vi "trajectory tracking.vi"() -> ()   [LabVIEW 2018]
doc: "Demonstrates the use of the Network Streams functions to send LED status to the myRIO target."
uses:
  <vilib>/addons/zeromq/socket_type.ctl
  <vilib>/ErrorRing/Error Ring.xnode
  <vilib>/vision/NI_Vision_Development_Module.lvlib
  <vilib>/addons/zeromq/zmq_socket.lvclass
  <vilib>/addons/zeromq/zmq_context.lvclass
  <vilib>/addons/zeromq/zeromq.lvlib
panel:
  out "u(t)_y":ext
  out "u(t)_x":ext
  out "relative_real_y_color":ext
  out "relative_real_x_color":ext
  in  "中心轨迹":bool
  in  "打开彩色点轨迹":bool
  out "relative_real_y_color":ext
  out "relative_real_x_color":ext
  out "彩色轨迹":T1(plugin-control)
  out "end_point_y":ext
  out "end_point_x":ext
  out "cy":ext
  out "cx":ext
  out "c":ext
  in  "簇 10":T2={"c"=100000.0, "cx"=100000.0, "cy"=100000.0, "start_point_x"=100000.0, "start_point_y"=100000.0}
  out "输出簇":T3
  in  "簇 9":T3={"a"=[], "b"=1.0, "a2"=[], "left1"=1.0, "top1"=1.0, "left2"=1.0, "top2"=1.0, "delta1"=1.0, "delta2"=1.0}
  in  "delta2":dbl=100.0
  out "bottom2":dbl
  out "right2":dbl
  out "top2":dbl
  out "left2":dbl
  in  "delta1":dbl=100.0
  out "bottom1":dbl
  out "right1":dbl
  out "top1":dbl
  out "left1":dbl
  out "delta_pr":dbl
  out "delta_dr":dbl
  in  "k2":dbl=-0.3
  in  "K1":dbl=0.3
  in  "Operation":T4(ring)=enum."Erode"
  out "old_real_relative_point_y":dbl
  out "old_real_relative_point_x":dbl
  out "real_relative_start_point_y":dbl
  out "real_relative_start_point_x":dbl
  out "Bounding Box.Y Top 2":i32
  out "Bounding Box.X Left 2":i32
  out "Ki part":dbl
  out "Kd part":dbl
  out "Kp part":dbl
  out "Ki part":dbl
  out "Kd part":dbl
  out "Kp part":dbl
  in  "Ki":dbl=0.0033
  in  "Kd":dbl=1e-05
  in  "Kp":dbl=0.01
  in  "Ki":dbl=0.0033
  in  "Kd":dbl=1e-05
  in  "Kp":dbl=0.01
  out "添加的数组":dbl[](array[numeric])
  out "desired_relative_point_y":dbl=820.0
  out "desired_relative_point_x":dbl=730.0
  out "MLP_pr":dbl=20.0
  out "MLP_dr":dbl=8.0
  out "error_relative_point_y":dbl
  out "error_relative_point_x":dbl
  out "real_relative_end_point_y":dbl
  out "real_relative_end_point_x":dbl
  out "magnet_input_pr":dbl
  out "magnet_input_dr":dbl
  in  "打开仅尖端轨迹":bool
  out "仅尖端轨迹":T1(plugin-control)
  out "Bounding Box.Y Top":i32
  out "Bounding Box.X Left":i32
  out "curve_min_y":dbl
  out "curve_min_x":dbl
  out "curve_max_y":dbl
  out "curve_max_x":dbl
  out "relative_end_point_y":dbl
  out "relative_end_point_x":dbl
  out "delta_y":dbl
  out "delta_x":dbl
  out "pr":dbl=-28.0
  out "tan(v)":dbl
  out "delta_velocity":dbl format="%#_10g"
  out "delta_time":dbl
  out "now time":timestamp[](array[timestamp])
  out "prev time":timestamp[](array[timestamp])
  out "delta_distance":dbl
  out "prev_end_point_y":dbl
  out "prev_end_point_x":dbl
  out "now_end_point_y":dbl
  out "now_end_point_x":dbl
  out "prev_end_point_y":dbl[](array[numeric])
  out "prev_end_point_x":dbl[](array[numeric])
  out "dr":dbl=120.0
  in  "Ar":sgl=11.0
  out "all parameters":dbl[][](array[numeric])
  out "direction angle":sgl[](array[numeric])
  out "dr":sgl
  out "strength":dbl[](array[numeric])
  out "场强":dbl
  out "end_point_y":T5
  out "end_point_x":dbl[](array[numeric])
  out "start_point_y":dbl[](array[numeric])
  out "start_point_x":dbl[](array[numeric])
  out "T":i32[](array[numeric])
  out "c":dbl[](array[numeric])
  out "b":dbl[](array[numeric])
  out "a\na":dbl[](array[numeric])
  out "c":dbl
  out "b":dbl
  out "a":dbl
  out "Angles (deg)":sgl[](array[numeric]) format="%.2f"
  in  "wr":sgl
  in  "打开轨迹":bool
  out "中心轨迹和尖端轨迹":T1(plugin-control)
  out "end_y":dbl
  out "end_x":dbl
  out "start_y":dbl
  out "start_x":dbl
  out "Image Pixels (U8)":u8[][](array[numeric])
  in  "Poly":dbl
  out "中心轨迹":T1(plugin-control)
  in  "保存按钮":bool
  out "Object Center":cluster{"X":sgl, "Y":sgl}
  out "黑白图":T1(plugin-control)
  in  "Number of Erosion":i32=5
  in  "Settings":T6={"Objects"=1, "Threshold"=128, "Reject Border"=FALSE, "Fill Holes"=FALSE, "Min Object Size"=TRUE, "Min Size"=1700, "Max Object Size"=FALSE, "Max Size"=100, "Show Search Area"=TRUE, "Show Center"=TRUE, "Show Bounding Box"=TRUE} {"Objects" items=["Bright Objects", "Dark Objects"]; "Threshold" min=1 max=999999999 step=1; "Max Size" min=1 max=999999999 step=1; "Min Size" min=1 max=999999999 step=1}
  out "Objects":T7(array[cluster]) {"Aspect Ratio" format="%.2f"; "Orientation" format="%.2f"; "Area" format="%.2f"; "Object Center"."Y" format="%.2f"; "Object Center"."X" format="%.2f"}
  in  "Search Rect (entire image)":T8={"Left"=350, "Top"=150, "Right"=1050, "Bottom"=1080, "Rotation"=0.0} {"Rotation" format="%.2f"; "Left" scale=0.0..1024.0; "Right" scale=0.0..1024.0}
  in  "Range":cluster{"Lower value":sgl, "Upper value":sgl}={"Lower value"=182.0, "Upper value"=255.0} {"Upper value" format="%.2f"; "Lower value" format="%.2f"}
  out "原图":T1(plugin-control)
  in  "停止":bool
  out "T":i32
  out "T":i32
  in  "磁场变换":bool=TRUE
  in  "Pause":bool
  out "Array":ext[](array[numeric])
  in  "Parameter Settings":T9(tab)=enum."Rotating Field" caption="Field Types"
  in  "Ag":dbl
  in  "dg":dbl
  in  "pg":dbl
  in  "fg":dbl
  in  "AoOF":dbl
  in  "fo":sgl
  in  "do":sgl
  in  "oo":sgl
  in  "po":sgl
  in  "cc":sgl
  in  "pc":sgl
  in  "wc":sgl
  in  "dc":sgl
  in  "Ac":dbl
  in  "Dis phase step":dbl
  in  "Dis phase frequency (Hz)":dbl
  in  "Dis tumbling frequency (Hz)":dbl
  in  "Dis strength(mT)":dbl
  in  "Swa strength (mT)":dbl
  in  "Swa frequency (Hz)":dbl
  in  "Swa pitch angle (deg)":dbl
  in  "Swa direction angle (deg)":dbl
  in  "Swa ratio":dbl=1.0
  in  "Pitch Angle (rotating around Constant, deg)":dbl
  in  "Ratio (A/C)":sgl
  in  "Direction Angle (deg)":sgl
  in  "Pitch Angle (rotating around Origin, deg)":sgl
  in  "Frequency (Hz)":sgl
  in  "Strength (mT)":dbl
  in  "Ar 2":dbl caption="Ar"
  in  "ratio":sgl
  in  "pr  2":sgl
  in  "dr  2":sgl
  in  "wr  2":sgl
  in  "p_x":sgl
  out "Numeric 5":i32
  in  "Stop":bool
  out "error out":errorcluster
  in  "Target IP Address":string="172.22.11.2"
  # "Overview: Magnetic field calculation, and send parameters to myRIO\nInstructions:\n1. Verify the value of Target IP Address. Set Visa resource name.\n2. Ensure RT Main.vi is already running. \n3. Run this VI. Set parameters of magnetic field."
  # "Strength (mT)"
  # "Frequency (Hz)"
  # "Pitch Angle (deg)"
  # "Direction Angle (deg)"
  # "Strength (mT)"
  # "Pitch Angle (deg)"
  # "Direction Angle (deg)"
  # "Frequency (Hz)"
  # "Strength (mT)"
  # "Oscilation Frequency (Hz)"
  # "Oscilation Angle (deg)"
  # "Pitch Angle (deg)"
  # "Direction Angle (deg)"
  # "Strength (mT)"
  # "Frequency (Hz)"
  # "Pitch Angle (deg)"
  # "Direction Angle (deg)"
  # "Conical Angle (deg)"
  # "Strength (mT)"
  # "Tumbling Frequency (Hz)"
  # "Phase Frequency (Hz)"
  # "Phase Step"
  # "Strength (mT)"
  # "Frequency (Hz)"
  # "Pitch Angle (deg)"
  # "Direction Angle (deg)"
  # "Ratio"
  # "Strength (mT)"
  # "Frequency (Hz)"
  # "Ratio (A/C)"
  # "Direction Angle (deg)"
  # "Pitch Angle (rotating around Origin, deg)"
  # "Pitch Angle (rotating around Constant, deg)"
  # "Strength (mT)"
  # "Frequency (Hz)"
  # "Pitch Angle Y (deg)"
  # "Pitch Angle X (deg)"
  # "Direction Angle (deg)"
  # "ratio (l/s)"
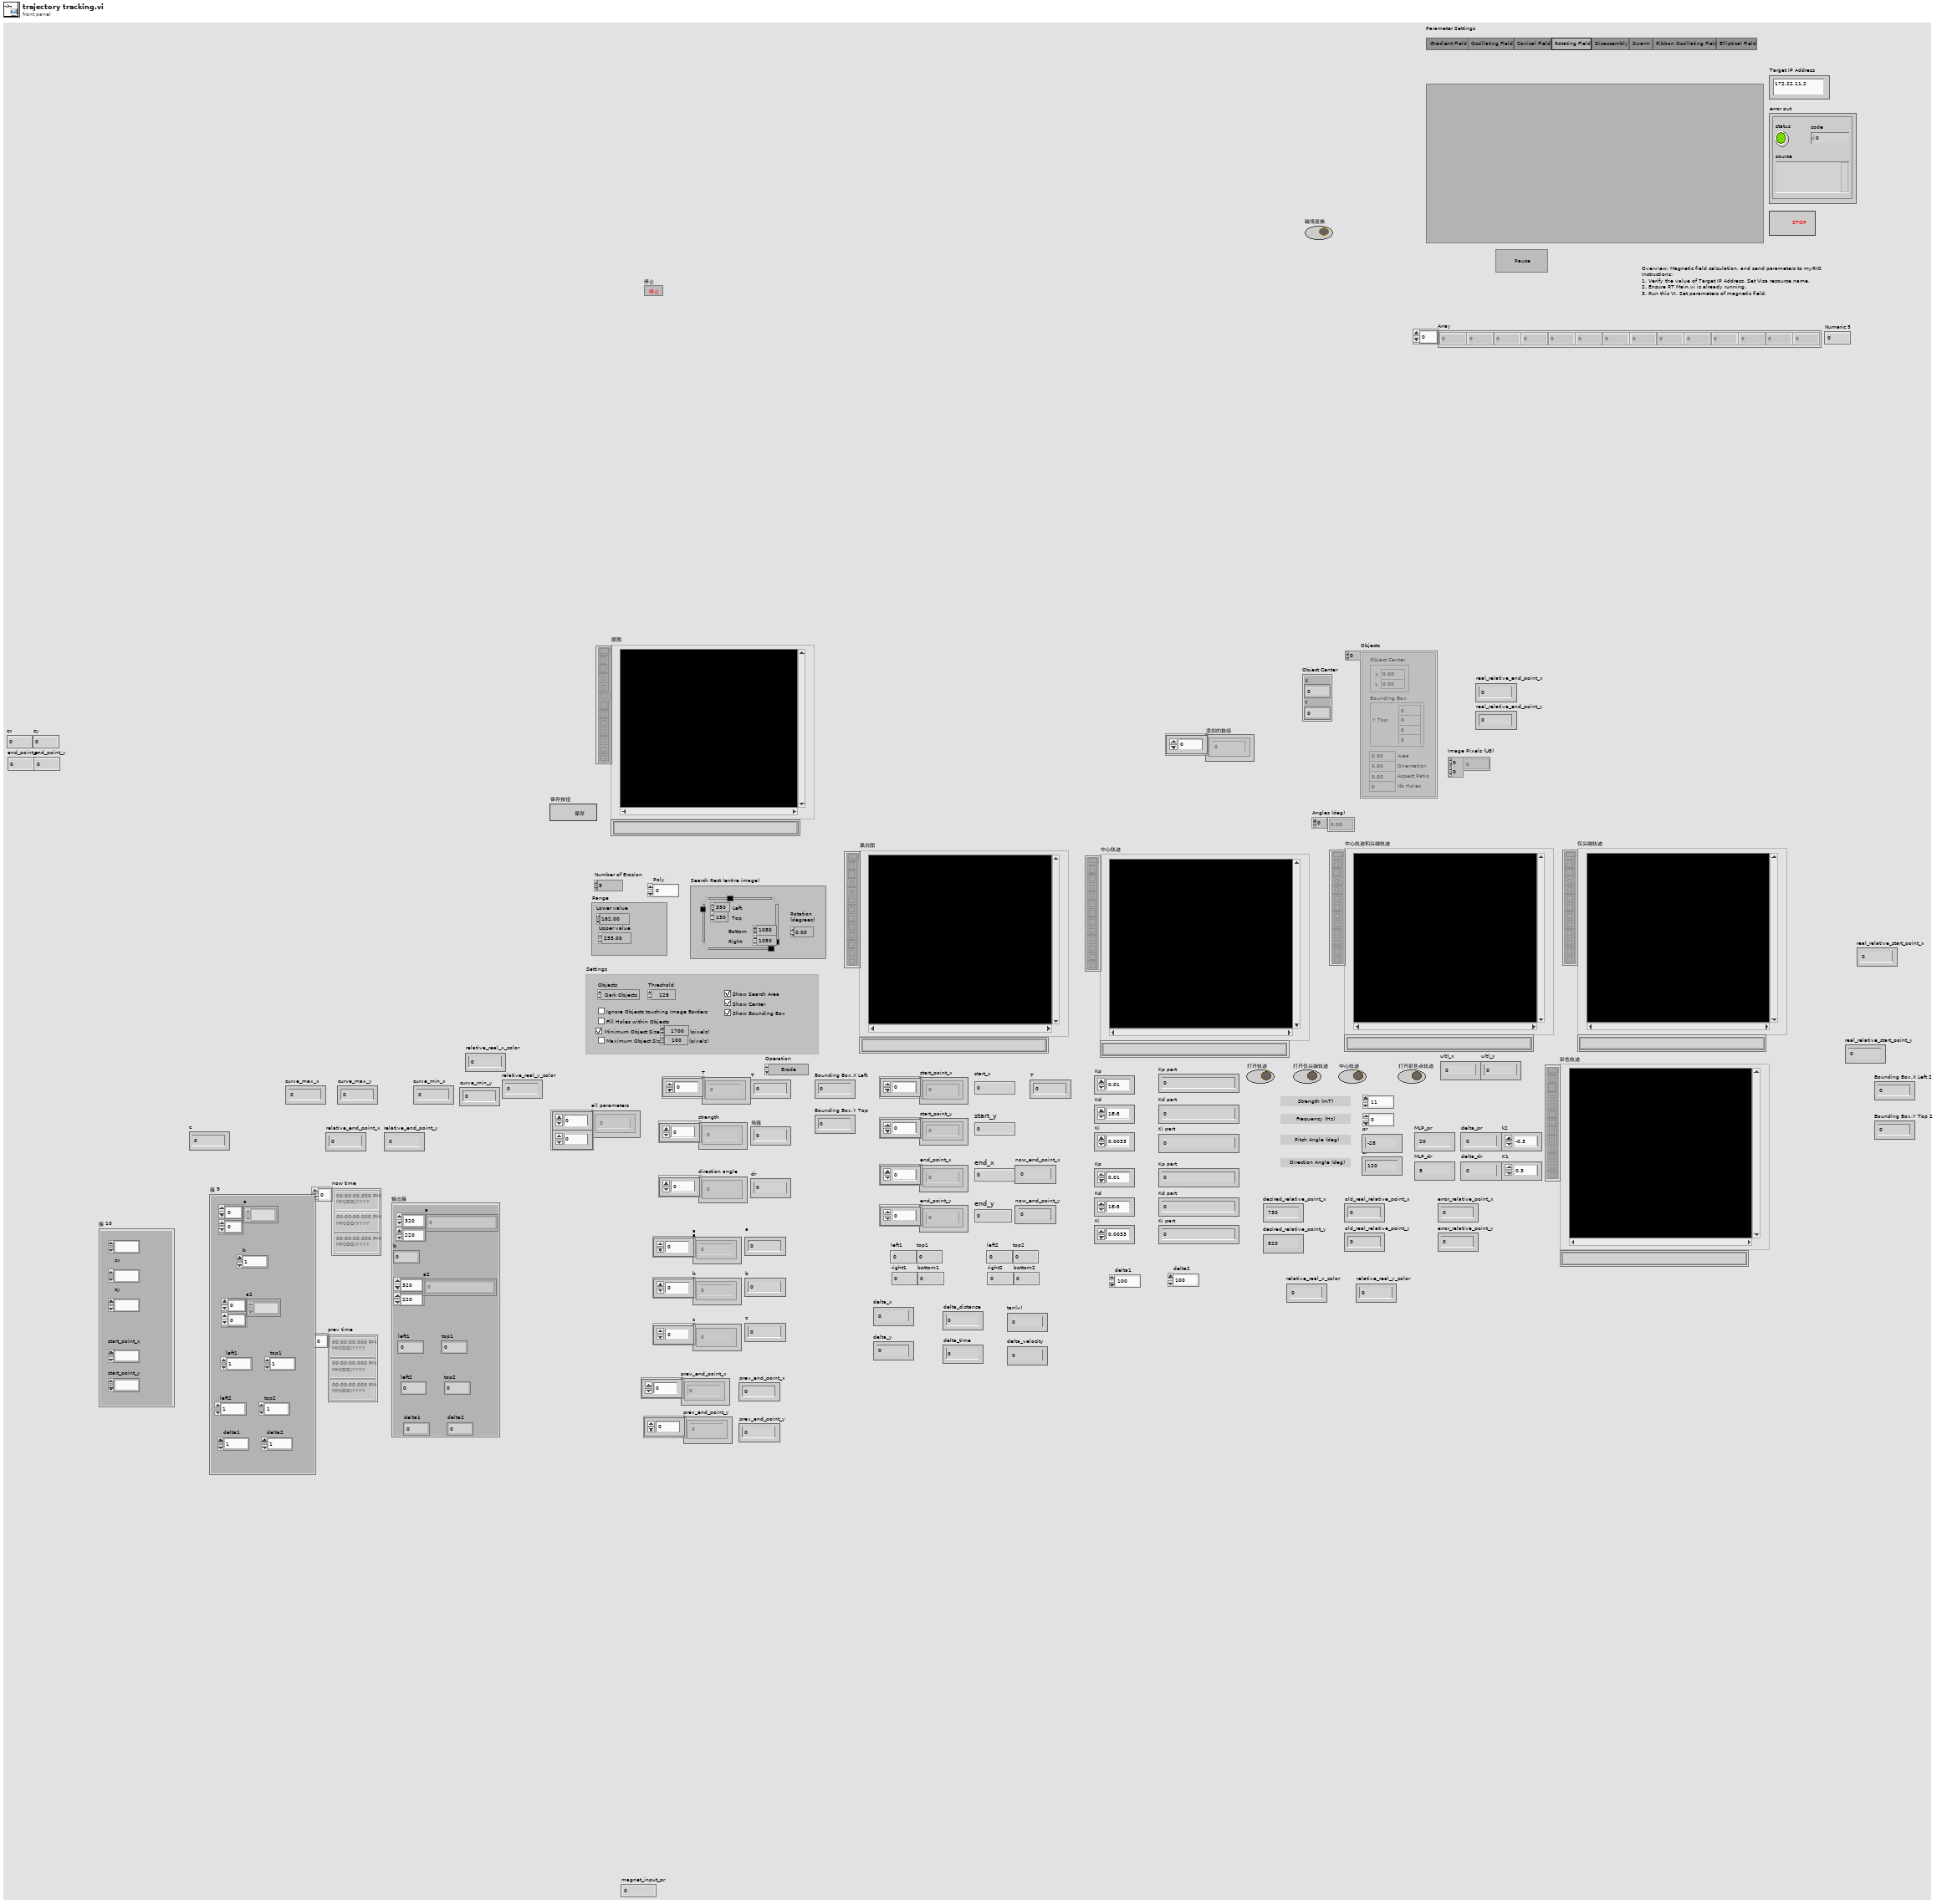
[diagram p1: front panel]
types:
  T1 = typedef "IMAQ Image.ctl" = refnum<image>
  T2 = cluster{"c":ext, "cx":ext, "cy":ext, "start_point_x":ext, "start_point_y":ext}
  T3 = cluster{"a":ext[][], "b":dbl, "a2":ext[][], "left1":dbl, "top1":dbl, "left2":dbl, "top2":dbl, "delta1":dbl, "delta2":dbl}
  T4 = enum32{"AutoM", "Close", "Dilate", "Erode", "Gradient", "Gradient in", "Gradient out", "HitMiss", "Open", "PClose", "POpen", "Thick", "Thin"}
  T5 = typedef "控件 3.ctl" = dbl[]
  T6 = cluster{"Objects":u16, "Threshold":i32, "Reject Border":bool, "Fill Holes":bool, "Min Object Size":bool, "Min Size":i32, "Max Object Size":bool, "Max Size":i32, "Show Search Area":bool, "Show Center":bool, "Show Bounding Box":bool}
  T7 = cluster{"Object Center":cluster{"X":sgl, "Y":sgl}, "Bounding Box":cluster{"X Left":i32, "Y Top":i32, "X Right":i32, "Y Bottom":i32}, "Area":sgl, "Orientation":sgl, "Aspect Ratio":sgl, "Nb Holes":i32}[]
  T8 = typedef "IMAQ Rectangle" = cluster{"Left":i32, "Top":i32, "Right":i32, "Bottom":i32, "Rotation":dbl}
  T9 = enum32{"Gradient Field ", "Oscillating Field", "Conical Field", "Rotating Field", "Disassembly", "Swarm", "Ribbon Oscillating Field", "Elliptical Field"}
  T10 = typedef "zeromq.lvlib/socket_type.ctl" = enum8{"ZMQ_PAIR", "ZMQ_PUB", "ZMQ_SUB", "ZMQ_REQ", "ZMQ_REP", "ZMQ_DEALER", "ZMQ_ROUTER", "ZMQ_PULL", "ZMQ_PUSH", "ZMQ_XPUB", "ZMQ_XSUB", "ZMQ_STREAM", "ZMQ_SERVER", "ZMQ_CLIENT", "ZMQ_RADIO", "ZMQ_DISH", "ZMQ_GATHER", "ZMQ_SCATTER", "ZMQ_DGRAM"}
  T11 = typedef "Image Type" = u32
  T12 = cluster{"Object Center":cluster{"X":sgl, "Y":sgl}, "Bounding Box":cluster{"X Left":i32, "Y Top":i32, "X Right":i32, "Y Bottom":i32}, "Area":sgl, "Orientation":sgl, "Aspect Ratio":sgl, "Nb Holes":i32}
  T13 = cluster{"X Left":i32, "Y Top":i32, "X Right":i32, "Y Bottom":i32, "Rotation":dbl}
  T14 = typedef "ROI Descriptor" = cluster{"Global Rectangle":i32[], "Contours":cluster{"ID":enum32{"External", "Internal"}, "Type":u32, "Coordinates":i32[]}[]}
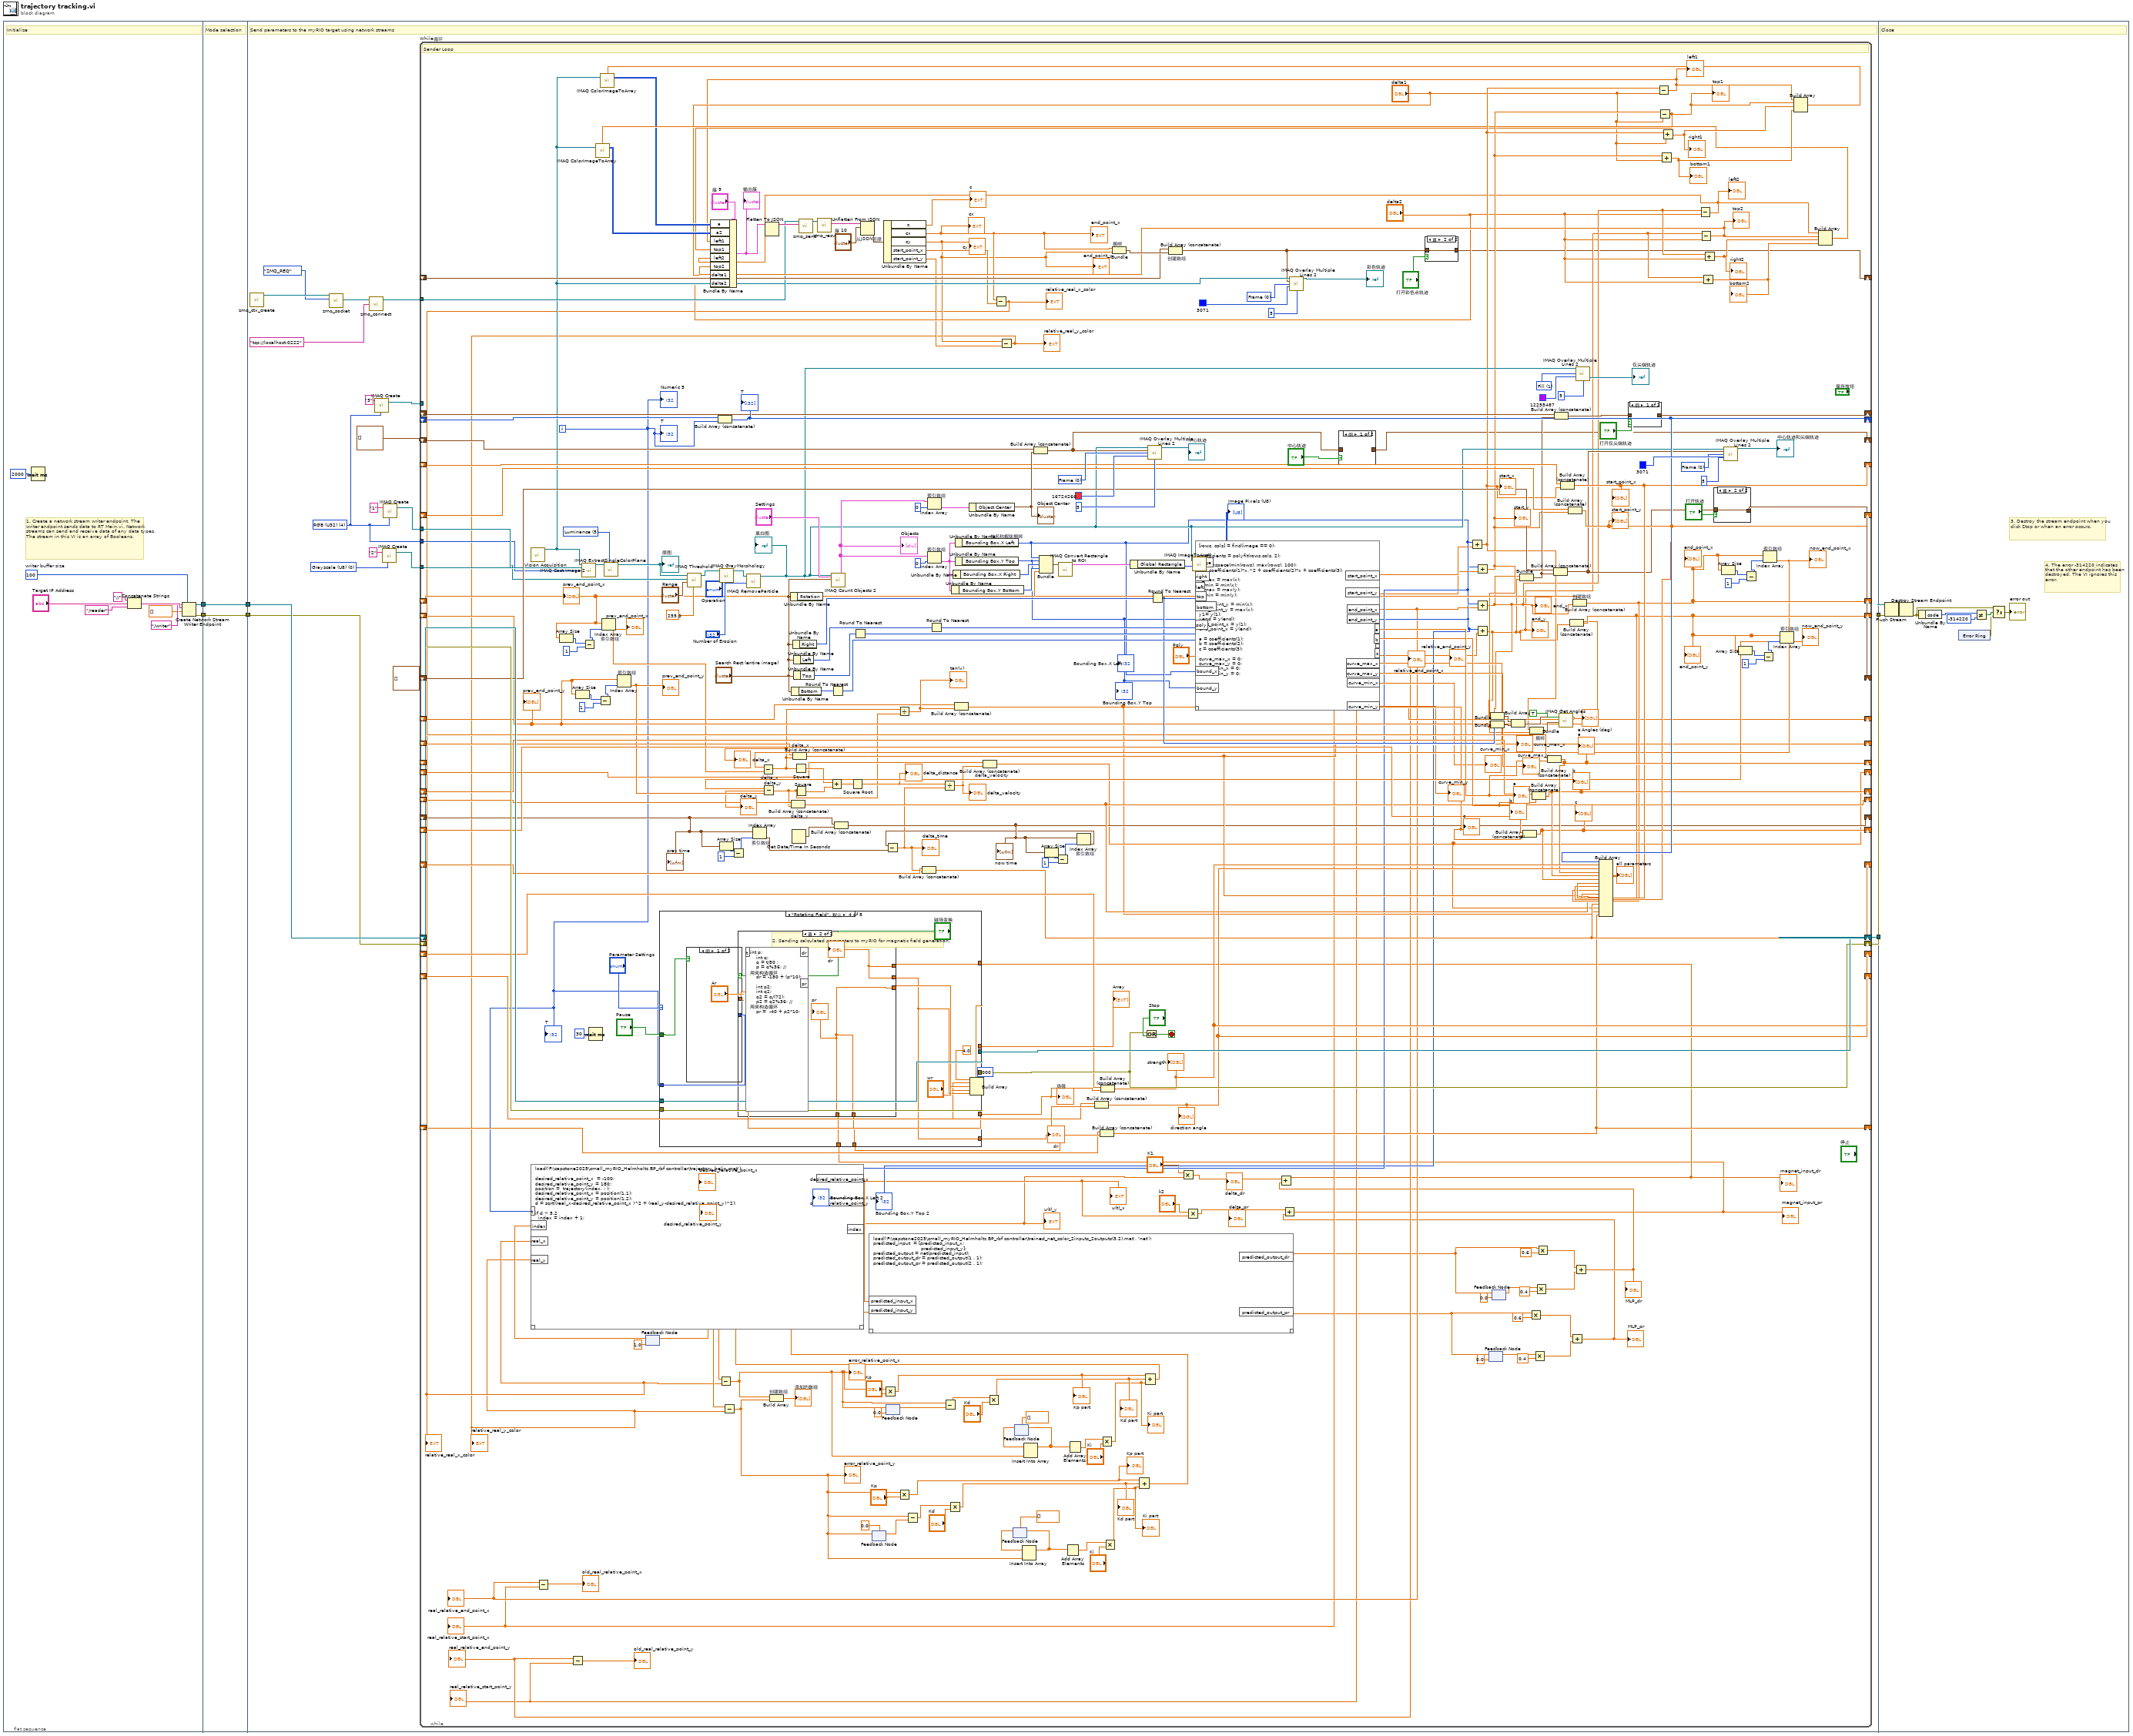
[diagram p0: block diagram]
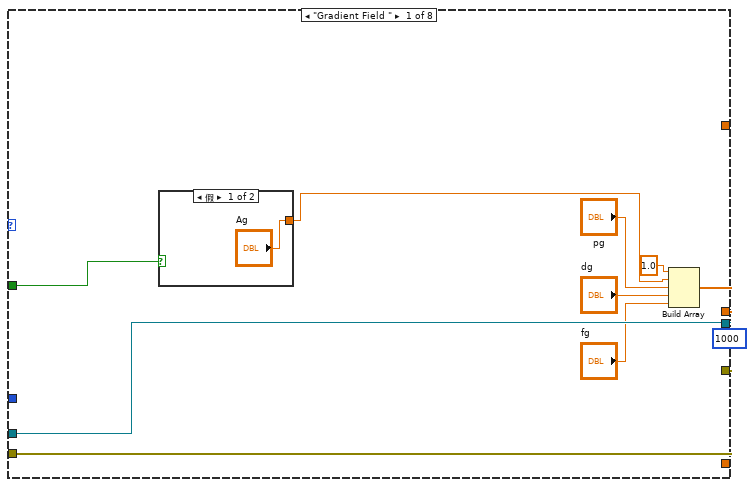
[diagram p6: hidden frame]
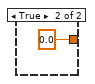
[diagram p7: hidden frame]
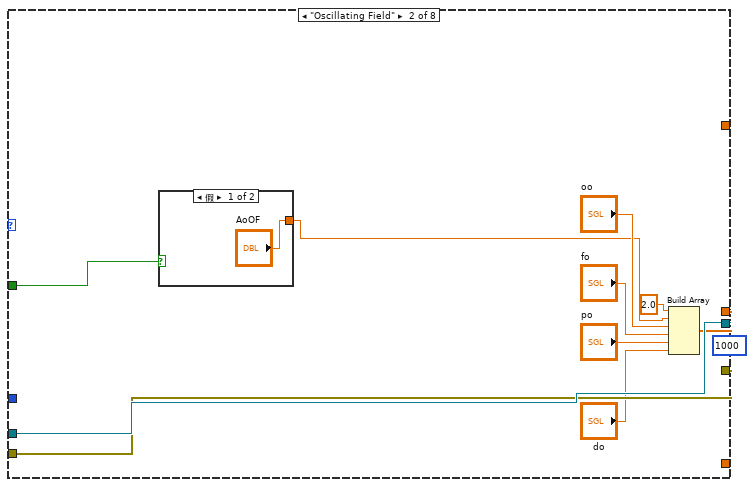
[diagram p8: hidden frame]
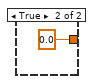
[diagram p9: hidden frame]
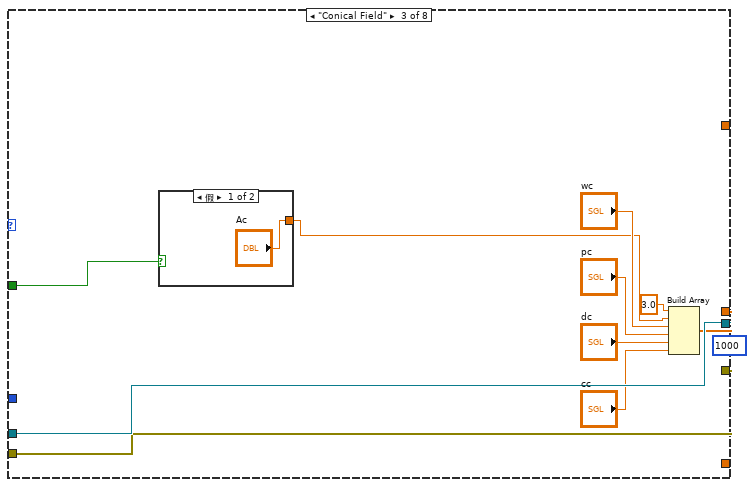
[diagram p10: hidden frame]
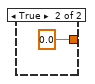
[diagram p11: hidden frame]
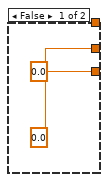
[diagram p12: hidden frame]
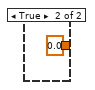
[diagram p13: hidden frame]
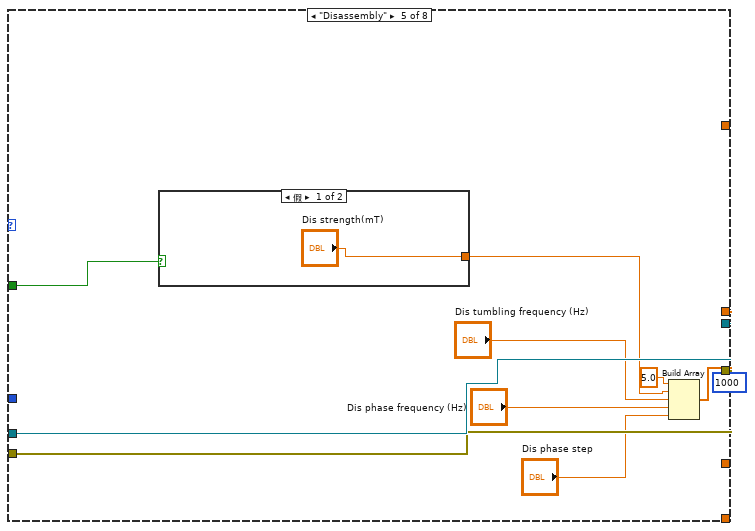
[diagram p14: hidden frame]
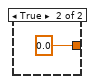
[diagram p15: hidden frame]
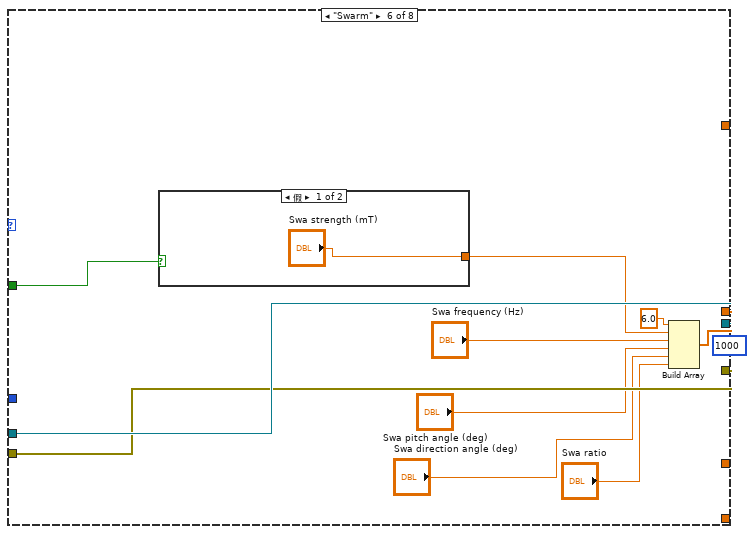
[diagram p16: hidden frame]
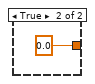
[diagram p17: hidden frame]
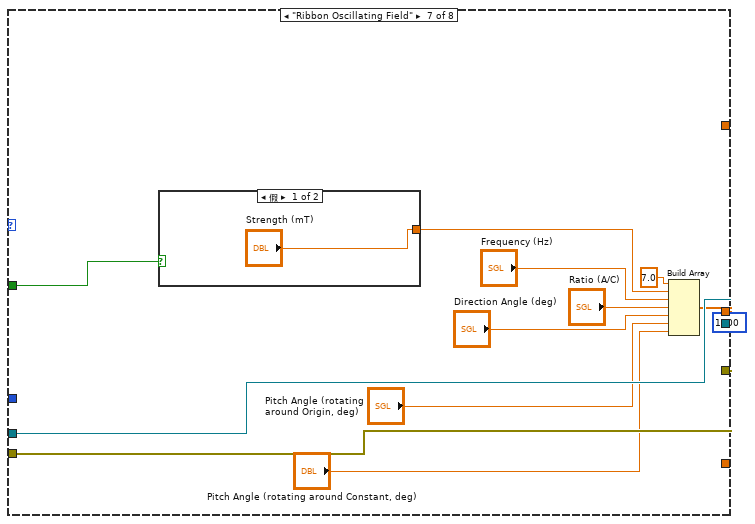
[diagram p18: hidden frame]
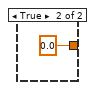
[diagram p19: hidden frame]
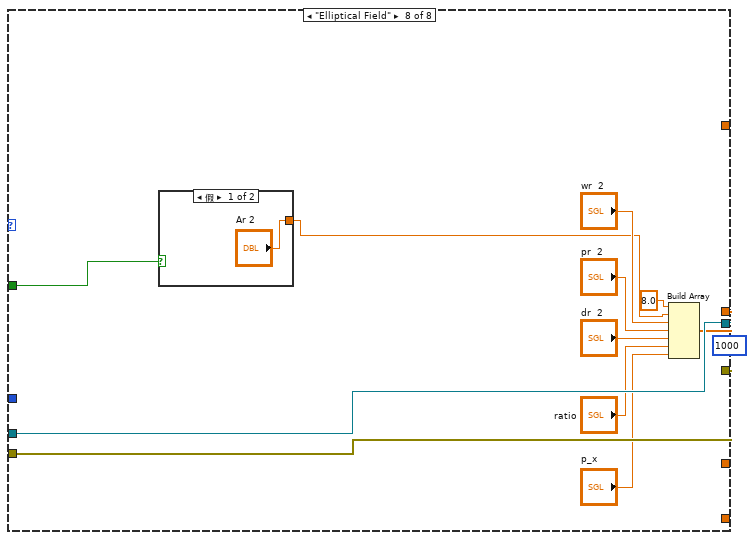
[diagram p20: hidden frame]
diagram:
  n1 = flat-sequence {
    tunnel: [w11] -> w2
    tunnel: [w10] -> w1
    tunnel: [w18] -> w4
    tunnel: [w17] -> w3
    tunnel: w1 -> [w17]
    tunnel: w2 -> [w18]
    tunnel: [w35] -> w6
    tunnel: w4 -> [w37]
    tunnel: [w34] -> w5
    tunnel: w3 -> [w36]
    tunnel: w6 -> [w447]
    tunnel: w5 -> [w444]
    frame #0 {
      w9 = 100  # writer buffer size
      # "1. Create a network stream writer endpoint. The writer endpoint sends data to RT Main.vi. Network streams can send and receive data of any data types. The stream in this VI is an array of Booleans."
      # "Initialize"
      n2 = Wait (ms)(milliseconds to wait=2000) -> ()  [unwired: 1 out]
      n3 = Concatenate Strings("//", "Target IP Address", "/reader") -> (w16:string)
      n4 = Create Network Stream Writer Endpoint(7:w9, 9:dbl[] [], 10:w16, 11:"/writer" ("reader name")) -> (0:w10:errorcluster, 3:w11:refnum<k21>)  [unwired: 3 in]
    }
    frame #1 {
      # "Mode selection"
    }
    frame #2 {
      w31 = T11 0 items=["Grayscale (U8)", "Grayscale (I16)", "Grayscale (SGL)", "Complex (CSG)", "RGB (U32)", "HSL (U32)", "RGB (U64)", "Grayscale (U16)"] ("Image Type")
      w24 = T11 4 items=["Grayscale (U8)", "Grayscale (I16)", "Grayscale (SGL)", "Complex (CSG)", "RGB (U32)", "HSL (U32)", "RGB (U64)", "Grayscale (U16)"] ("Image Type")
      # "Send parameters to the myRIO target using network streams"
      n5 = call <vilib>:"zmq_ctx_create.vi"() -> ("context out"=w22:refnum<class "zmq_context.lvclass">)  [unwired: 4 in, 1 out]
      n6 = call <vilib>:"zmq_socket.vi"("socket type"=socket_type."ZMQ_REQ", "context in"=w22) -> ("socket out"=w23:refnum<class "zmq_socket.lvclass">)  [unwired: 3 in, 2 out]
      n7 = call <vilib>:"zmq_connect.vi"("endpoint"="tcp://localhost:0222", "socket in"=w23) -> ("socket out"=w19:refnum<class "zmq_socket.lvclass">)  [unwired: 2 in, 1 out]
      n8 = call "IMAQ Create"("Image Name"="3", "Image Type"=w24) -> ("New Image"=w27:T1)  [unwired: 3 in, 1 out]
      n9 = call "IMAQ Create"("Image Name"="2", "Image Type"=w31) -> ("New Image"=w29:T1)  [unwired: 3 in, 1 out]
      n10 = call "IMAQ Create"("Image Name"="1", "Image Type"=w24) -> ("New Image"=w30:T1)  [unwired: 3 in, 1 out]
      n11 = while "While循环" {
        shift-right: [w300] -> w34
        shift-left: w36 -> [w302]
        shift-right: [w301] -> w35
        shift-left: w37 -> [w303]
        tunnel: w30 -> [w256]
        tunnel: w29 -> [w255]
        tunnel: w27 -> [_]
        shift-right: [w252] -> _
        shift-left: cluster{"X":dbl, "Y":dbl}[] [] -> [w257]
        shift-right: [w44] -> _
        shift-left: cluster{"X":dbl, "Y":dbl}[] [] -> [w258]
        tunnel: w24 -> [w254]
        shift-right: [w228] -> _
        shift-left: _ -> [w244]
        shift-right: [w223] -> _
        shift-left: _ -> [w242]
        shift-right: [w227] -> _
        shift-left: _ -> [w239]
        shift-right: [w231] -> _
        shift-left: _ -> [w238]
        shift-right: [w226] -> _
        shift-left: _ -> [w237]
        shift-right: [w225] -> _
        shift-left: _ -> [w236]
        shift-right: [w219] -> _
        shift-left: _ -> [w211]
        shift-right: [w215] -> _
        shift-left: _ -> [w207]
        shift-right: [w230] -> _
        shift-left: _ -> [w234]
        shift-right: [w229] -> _
        shift-left: _ -> [w232]
        shift-right: [w196] -> _
        shift-left: _ -> [w198]
        shift-right: [w195] -> _
        shift-left: _ -> [w197]
        shift-right: [w185] -> _
        shift-left: _ -> [w190]
        shift-right: [w182] -> _
        shift-left: _ -> [w183]
        shift-right: [w178] -> _
        shift-left: _ -> [w179]
        shift-right: [w173] -> _
        shift-left: _ -> [w174]
        shift-right: [w165] -> _
        shift-left: _ -> [w166]
        shift-right: [w159] -> _
        shift-left: _ -> [w160]
        shift-right: [w48] -> _
        shift-left: _ -> [w65]
        tunnel: w19 -> [w63]
        i -> [w153]
        stop <- w296 stop-if-true
        w73 = u32 0 items=["Frame", "Fill"] ("Drawing Mode (Frame)")
        w161 = u32 1 items=["Frame", "Fill"] ("Drawing Mode (Frame)")
        w168 = u32 0 items=["Frame", "Fill"] ("Drawing Mode (Frame)")
        w283 = u32 0 items=["Frame", "Fill"] ("Drawing Mode (Frame)")
        w293 = 5 items=["Red", "Green", "Blue", "Hue", "Saturation", "Luminance", "Value", "Intensity"] ("Color Plane")
        # "2. Sending calculated parameters to myRIO for magnetic field generation."
        # "Sender Loop"
        n12 = call "Vision Acquisition"() -> ("Image Out"=w62:T1)  [unwired: 23 in, 4 out]
        n13 = Array Size(array=w211) -> (size(s)=w213:i32)
        n14 = Array Size(array=w207) -> (size(s)=w209:i32)
        n15 = call "IMAQ Cast Image 2"("Image Src"=w62, "Image Dst"=w256, "Image Type"=w254) -> ("Image Dst Out"=w294:T1)  [unwired: 11 in, 1 out]
        n16 = Subtract(x=w213, y=1) -> (x-y=w212:i32)
        n17 = Wait (ms)(milliseconds to wait=u32 30 ("等待时间（毫秒）")) -> ()  [unwired: 1 out]
        n18 = Subtract(x=w209, y=1) -> (x-y=w208:i32)
        n19 = Index Array "索引数组"(array=w211, index=w212) -> (element=w205:dbl)
        "prev_end_point_x" <- w205
        n20 = call "IMAQ ExtractSingleColorPlane"("Color Plane"=w293, "Image Src"=w294) -> ("Image Dst Out"=w292:T1)  [unwired: 8 in, 1 out]
        "原图" <- w292
        n21 = Index Array "索引数组"(array=w207, index=w208) -> (element=w204:dbl)
        "prev_end_point_y" <- w204
        n22 = feedback #1(1.0) -> (w59:dbl)
        n23 = call "IMAQ Threshold"("Replace Value"=sgl 255.0, "Range"="Range", "Image Dst"=w255, "Image Src"=w292) -> ("Image Dst Out"=w117:T1)  [unwired: 6 in, 1 out]
        n24 = Build Array (concatenate)(w238, w153) -> (w231:i32[])
        "T" <- w231
        n25 = call "IMAQ GrayMorphology"("Operation"="Operation", "Image Src"=w117) -> ("Image Dst Out"=w116:T1)  [unwired: 8 in, 1 out]
        n26 = Array Size(array=w190) -> (size(s)=w193:i32)
        n27 = Subtract(x=w193, y=1) -> (x-y=w192:i32)
        n28 = call "IMAQ RemoveParticle"("Number of Erosion"="Number of Erosion", "Image Src"=w116) -> ("Image Dst Out"=w157:T1)  [unwired: 8 in, 1 out]
        "黑白图" <- w157
        n29 = Index Array "索引数组"(array=w190, index=w192) -> (element=w189:timestamp)
        n30 = Unbundle By Name("Search Rect (entire image)") -> ("Rotation"=w279:dbl)
        n31 = Unbundle By Name("Search Rect (entire image)") -> ("Bottom"=w263:i32)
        n32 = Get Date/Time In Seconds() -> (seconds since 1Jan1904=w194:timestamp)
        n33 = Unbundle By Name("Search Rect (entire image)") -> ("Right"=w267:i32)
        n34 = Unbundle By Name("Search Rect (entire image)") -> ("Left"=w266:i32)
        n35 = Unbundle By Name("Search Rect (entire image)") -> ("Top"=w265:i32)
        n36 = Round To Nearest(number=w263) -> (nearest integer value=w262:i32)
        n37 = call "IMAQ Count Objects 2"("Settings"="Settings", "Search Rect (entire image)"="Search Rect (entire image)", "Image"=w157) -> ("Objects"=w281:T7)  [unwired: 4 in, 4 out]
        "Objects" <- w281
        n38 = Build Array (concatenate)(w190, w194) -> (w185:timestamp[])
        "now time" <- w185
        n39 = Round To Nearest(number=w265) -> (nearest integer value=w264:i32)
        n40 = feedback #2(0.0) -> (w135:ext)
        n41 = feedback #3(0.0) -> (w149:ext)
        n42 = Index Array "索引数组"(array=w281, index=0 ("索引")) -> (element=w286:T12)
        n43 = Index Array "索引数组"(array=w281, index=0 ("索引")) -> (element=w277:T12)
        n44 = Round To Nearest(number=w266) -> (nearest integer value=w260:i32)
        n45 = Unbundle By Name(w277) -> ("Bounding Box.Y Bottom"=w271:i32)
        n46 = Unbundle By Name(w277) -> ("Bounding Box.X Right"=w272:i32)
        n47 = Unbundle By Name "按名称解除捆绑"(w277) -> ("Bounding Box.X Left"=w123:i32)
        "Bounding Box.X Left" <- w123
        "Bounding Box.X Left 2" <- w123
        n48 = Unbundle By Name(w277) -> ("Bounding Box.Y Top"=w122:i32)
        "Bounding Box.Y Top" <- w122
        "Bounding Box.Y Top 2" <- w122
        n49 = Unbundle By Name(w286) -> ("Object Center"=w285:cluster{"X":sgl, "Y":sgl})
        "Object Center" <- w285
        n50 = feedback #4(dbl[] []) -> (w130:dbl[])
        n51 = feedback #5(dbl[] []) -> (w144:dbl[])
        n52 = Build Array (concatenate)(w258, w285) -> (w45:cluster{"X":dbl, "Y":dbl}[])
        n53 = Bundle("X Left"=w123, "Y Top"=w122, "X Right"=w272, "Y Bottom"=w271, "Rotation"=w279) -> (w278:T13)  [unwired: 1 in]
        n54 = Array Size(array=w185) -> (size(s)=w188:i32)
        n55 = Subtract(x=w188, y=1) -> (x-y=w187:i32)
        n56 = call "IMAQ Convert Rectangle to ROI"("Rectangle"=w278) -> ("ROI Descriptor"=w276:T14)  [unwired: 8 in, 1 out]
        n57 = Index Array "索引数组"(array=w185, index=w187) -> (element=w184:timestamp)
        n58 = Subtract(x=w184, y=w189) -> (x-y=w181:dbl)
        "delta_time" <- w181
        n59 = Build Array (concatenate)(w183, w181) -> (w182:dbl[])
        n60 = Unbundle By Name(w276) -> ("Global Rectangle"=w261:i32[])
        n61 = call "IMAQ Overlay Multiple Lines 2"("Image"=w157, "Line End Points"=w45, "Drawing Mode (Frame)"=w283, "Color"=u32 16724266, "Width"=u32 5) -> ("Image Out"=→"中心轨迹":T1)  [unwired: 9 in, 1 out]
        n62 = Round To Nearest(number=w267) -> (nearest integer value=w245:i32)
        n63 = call "IMAQ ImageToArray"("Optional Rectangle"=w261, "Image"=w157) -> ("Image Pixels (U8)"=w273:u8[][])  [unwired: 2 in, 4 out]
        "Image Pixels (U8)" <- w273
        n64 = script code="[rows, cols] = find(image == 0); \n\ncoefficients = polyfit(rows,cols, 2);\n\nx = linspace(min(rows), max(rows), 100); \ny = coefficients(1)*x.^2 + coefficients(2)*x + coefficients(3);\n\nx_max = max(x);\nx_min = min(x);\ny_max = max(y);\ny_min = min(y);\n\nstart_point_y = min(x);\nend_point_y = max(x);\ny1= y(1);\nyend = y(end);\nstart_point_x = y(1);\nend_point_x = y(end);\n\na = coefficients(1);\nb = coefficients(2);\nc = coefficients(3);\n\ncurve_max_x = 0;\ncurve_max_y = 0;\ncurve_min_x = 0;\ncurve_min_y = 0;"("image"=w273, "poly"="Poly", "right"=w245, "left"=w260, "top"=w264, "bottom"=w262, "bound_x"=w123, "bound_y"=w122) -> ("start_point_x"=w120:dbl, "start_point_y"=w118:dbl, "end_point_x"=w121:dbl, "end_point_y"=w119:dbl, "a"=w243:dbl, "b"=w241:dbl, "c"=w240:dbl, "curve_max_x"=→"curve_max_x":dbl, "curve_max_y"=→"curve_max_y":dbl, "curve_min_x"=→"curve_min_x":dbl, "curve_min_y"=→"curve_min_y":dbl)  [unwired: 1 in, 1 out]
        "a" <- w243
        "b" <- w241
        "c" <- w240
        "relative_end_point_x" <- w121
        "relative_end_point_y" <- w119
        "real_relative_end_point_x" <- w121
        "real_relative_end_point_y" <- w119
        "real_relative_start_point_x" <- w120
        "real_relative_start_point_y" <- w118
        n65 = Subtract(x=w121, y=w120) -> (x-y=→"old_real_relative_point_x":dbl)
        n66 = Subtract(x=w119, y=w118) -> (x-y=→"old_real_relative_point_y":dbl)
        n67 = case shown="假" "中心轨迹" {
          tunnel: w45 -> [_ w305]
          tunnel: [_ w305] -> w44
          frame False {
          }
          frame True {
          }
        }
        n68 = Add(x=w123, y=w120) -> (x+y=w88:dbl)
        "start_x" <- w88
        n69 = Add(x=w122, y=w118) -> (x+y=w87:dbl)
        "start_y" <- w87
        n70 = Add(x=w123, y=w121) -> (x+y=w86:dbl)
        "end_x" <- w86
        n71 = Add(x=w122, y=w119) -> (x+y=w85:dbl)
        "end_y" <- w85
        n72 = feedback #6(0.0) -> (w104:dbl)
        n73 = Bundle(w86, w85) -> (w249:cluster{dbl, dbl})  [unwired: 1 in]
        n74 = Bundle(w245, w87) -> (w248:cluster{i32, dbl})  [unwired: 1 in]
        n75 = feedback #7(0.0) -> (w112:dbl)
        n76 = Build Array(w249, w248) -> (w247:cluster{dbl, dbl}[])
        n77 = Bundle(w86, w85) -> (w155:cluster{dbl, dbl})  [unwired: 1 in]
        n78 = Build Array (concatenate)(w239, w240) -> (w227:dbl[])
        "c" <- w227
        n79 = Bundle "捆绑"(w88, w87) -> (w250:cluster{dbl, dbl})  [unwired: 1 in]
        n80 = Build Array (concatenate)(w242, w241) -> (w223:dbl[])
        "b" <- w223
        n81 = Multiply(x=w104, y=0.4) -> (x*y=w101:dbl)
        n82 = Multiply(x=w112, y=0.4) -> (x*y=w108:dbl)
        n83 = Build Array (concatenate)(w244, w243) -> (w228:dbl[])
        "a\na" <- w228
        n84 = Build Array (concatenate)(w257, w155) -> (w156:cluster{"X":dbl, "Y":dbl}[])
        n85 = Build Array (concatenate)(w160, w155) -> (w154:cluster{dbl, dbl}[])
        n86 = call "IMAQ Get Angles"("Vertex"=w250, "Points"=w247, "Use Vertex (No)"=TRUE) -> ("Angles (deg)"=→"Angles (deg)":sgl[])  [unwired: 2 in, 2 out]
        n87 = Build Array (concatenate)(w237, w88) -> (w226:dbl[])
        "start_point_x" <- w226
        n88 = Build Array (concatenate)(w236, w87) -> (w225:dbl[])
        "start_point_y" <- w225
        n89 = Build Array (concatenate)(w207, w85) -> (w215:dbl[])
        "end_point_y" <- w215
        n90 = Build Array (concatenate) "创建数组"(w211, w86) -> (w219:dbl[])
        "end_point_x" <- w219
        n91 = call "IMAQ Overlay Multiple Lines 2"("Image"=w157, "Drawing Mode (Frame)"=w161, "Color"=u32 12255487, "Width"=u32 5) -> ("Image Out"=→"仅尖端轨迹":T1)  [unwired: 10 in, 1 out]
        n92 = case shown="假" "打开仅尖端轨迹" {
          tunnel: [_ w307] -> w159
          tunnel: w154 -> [_ w307]
          frame False {
          }
          frame True {
          }
        }
        n93 = Subtract(x=w88, y="delta1") -> (x-y=w68:dbl)
        "left1" <- w68
        n94 = Subtract(x=w87, y="delta1") -> (x-y=w67:dbl)
        "top1" <- w67
        n95 = Add(x=w87, y="delta1") -> (x+y=w89:dbl)
        "bottom1" <- w89
        n96 = Add(x=w88, y="delta1") -> (x+y=w90:dbl)
        "right1" <- w90
        n97 = Subtract(x=w86, y="delta2") -> (x-y=w66:dbl)
        "left2" <- w66
        n98 = Subtract(x=w85, y="delta2") -> (x-y=w64:dbl)
        "top2" <- w64
        n99 = Add(x=w85, y="delta2") -> (x+y=w91:dbl)
        "bottom2" <- w91
        n100 = Add(x=w86, y="delta2") -> (x+y=w92:dbl)
        "right2" <- w92
        n101 = case shown="真" "打开轨迹" {
          tunnel: [_ w308] -> w252
          tunnel: w156 -> [_ w308]
          frame False {
          }
          frame True {
          }
        }
        n102 = Array Size(array=w219) -> (size(s)=w221:i32)
        n103 = call "IMAQ Overlay Multiple Lines 2"("Image"=w157, "Line End Points"=w156, "Drawing Mode (Frame)"=w168, "Color"=u32 3071, "Width"=u32 5) -> ("Image Out"=→"中心轨迹和尖端轨迹":T1)  [unwired: 9 in, 1 out]
        n104 = Array Size(array=w215) -> (size(s)=w217:i32)
        n105 = Subtract(x=w221, y=1) -> (x-y=w220:i32)
        n106 = Subtract(x=w217, y=1) -> (x-y=w216:i32)
        n107 = Index Array "索引数组"(array=w219, index=w220) -> (element=w206:dbl)
        "now_end_point_x" <- w206
        n108 = Subtract "delta_x"(x=w206, y=w205) -> (x-y=w177:dbl)
        "delta_x" <- w177
        n109 = Build Array (concatenate) "delta_x"(w198, w177) -> (w196:dbl[])
        n110 = Square(x=w177) -> (x^2=w202:dbl)
        n111 = Index Array "索引数组"(array=w215, index=w216) -> (element=w203:dbl)
        "now_end_point_y" <- w203
        n112 = Subtract "delta_y"(x=w203, y=w204) -> (x-y=w176:dbl)
        "delta_y" <- w176
        n113 = Build Array (concatenate) "delta_y"(w197, w176) -> (w195:dbl[])
        n114 = Square(x=w176) -> (x^2=w201:dbl)
        n115 = Add(x=w202, y=w201) -> (x+y=w200:dbl)
        n116 = Square Root(x=w200) -> (sqrt(x)=w199:dbl)
        "delta_distance" <- w199
        n117 = Divide(x=w177, y=w176) -> (x/y=w175:dbl)
        "tan(v)" <- w175
        n118 = Divide(x=w199, y=w181) -> (x/y=w180:dbl)
        "delta_velocity" <- w180
        n119 = Build Array (concatenate)(w174, w175) -> (w173:dbl[])
        n120 = Build Array (concatenate) "delta_velocity"(w179, w180) -> (w178:dbl[])
        n121 = Build Array(w68, w67, w90, w89) -> (w84:dbl[])
        n122 = call "IMAQ ColorImageToArray"("Optional Rectangle"=w84, "Image"=w62) -> ("Image Pixels (U32)"=w70:u32[][])  [unwired: 2 in, 2 out]
        n123 = Build Array(w66, w64, w92, w91) -> (w83:dbl[])
        n124 = call "IMAQ ColorImageToArray"("Optional Rectangle"=w83, "Image"=w62) -> ("Image Pixels (U32)"=w69:u32[][])  [unwired: 2 in, 2 out]
        n125 = Bundle By Name(cluster="簇 9", "a"=w70, "a2"=w69, "left1"=w68, "top1"=w67, "left2"=w66, "top2"=w64, "delta1"="delta1", "delta2"="delta2") -> (w76:T3)
        "输出簇" <- w76
        n126 = Flatten To JSON(anything=w76) -> (JSON string=w75:string)  [unwired: 2 in, 1 out]
        n127 = call <vilib>:"zmq_send.vi"("data"=w75, "socket in"=w63) -> ("socket out"=w80:refnum<class "zmq_socket.lvclass">)  [unwired: 5 in, 1 out]
        n128 = call <vilib>:"zmq_recv.vi"("socket in"=w80) -> ("data"=w81:string)  [unwired: 4 in, 4 out]
        n129 = Unflatten From JSON "从JSON还原"(JSON string=w81, type and defaults="簇 10") -> (value=w78:T2)  [unwired: 5 in, 1 out]
        n130 = Unbundle By Name(w78) -> ("c"=→"c":ext, "cx"=w53:ext, "cy"=w51:ext, "start_point_x"=w52:ext, "start_point_y"=w50:ext)
        "cx" <- w53
        "cy" <- w51
        "end_point_x" <- w53
        "end_point_y" <- w51
        n131 = Subtract(x=w53, y=w52) -> (x-y=w41:ext)
        "relative_real_x_color" <- w41
        "relative_real_x_color" <- w41
        n132 = Subtract(x=w51, y=w50) -> (x-y=w40:ext)
        "relative_real_y_color" <- w40
        "relative_real_y_color" <- w40
        n133 = script code="load('F:\\capstone2025\\small_myRIO_Helmholtz BP_rbf controller\\trajectory_helix.mat');\n\ndesired_relative_point_x  = -100;\ndesired_relative_point_y = 180;\nposition =  trajectory(index, : );\ndesired_relative_point_x = position(1,1);\ndesired_relative_point_y = position(1,2);\nd = sqrt((real_x-desired_relative_point_x )^2 + (real_y-desired_relative_point_y)^2);\n\nif d < 5.2\n  index = index + 1; \nend"("t"=w153, "index"=w59, "real_x"=w41, "real_y"=w40) -> ("desired_relative_point_x"=w43:dbl, "desired_relative_point_y"=w42:dbl, "index"=w60:dbl)  [unwired: 1 in, 1 out]
        "desired_relative_point_x" <- w43
        "desired_relative_point_y" <- w42
        n134 = feedback-in #1(w60) -> ()
        n135 = Subtract(x=w43, y=w41) -> (x-y=w143:ext)
        "error_relative_point_x" <- w143
        n136 = Subtract(x=w42, y=w40) -> (x-y=w128:ext)
        "error_relative_point_y" <- w128
        n137 = Build Array "创建数组"(w143, w128) -> (→"添加的数组":ext[])
        n138 = script code="load('F:\\capstone2025\\small_myRIO_Helmholtz BP_rbf controller\\trained_net_color_2inputs_2outputs(3,2).mat', 'net');\npredicted_input  = [predicted_input_x; \n                               predicted_input_y];\npredicted_output = net(predicted_input);\npredicted_output_dr = predicted_output(1 , 1);\npredicted_output_pr = predicted_output(2 , 1);"("predicted_input_y"=w42, "predicted_input_x"=w43) -> ("predicted_output_dr"=w113:dbl, "predicted_output_pr"=w106:dbl)  [unwired: 1 in, 1 out]
        n139 = feedback-in #2(w128) -> ()
        n140 = Multiply(x=w143, y="Kp") -> (x*y=w150:ext)
        "Kp part" <- w150
        n141 = feedback-in #3(w143) -> ()
        n142 = Multiply(x=w128, y="Kp") -> (x*y=w136:ext)
        "Kp part" <- w136
        n143 = Subtract(x=w128, y=w135) -> (x-y=w133:ext)
        n144 = Subtract(x=w143, y=w149) -> (x-y=w147:ext)
        n145 = Multiply(x=w133, y="Kd") -> (x*y=w131:ext)
        "Kd part" <- w131
        n146 = Multiply(x=w147, y="Kd") -> (x*y=w145:ext)
        "Kd part" <- w145
        n147 = Insert Into Array(array=w130, new element=w128) -> (w129:dbl[])  [unwired: 1 in]
        n148 = feedback-in #4(w129) -> ()
        n149 = Insert Into Array(array=w144, new element=w143) -> (w142:dbl[])  [unwired: 1 in]
        n150 = feedback-in #5(w142) -> ()
        n151 = Add Array Elements(numeric array=w129) -> (sum=w126:dbl)
        n152 = Add Array Elements(numeric array=w142) -> (sum=w140:dbl)
        n153 = Multiply(x=w140, y="Ki") -> (x*y=w138:dbl)
        "Ki part" <- w138
        n154 = Multiply(x=w126, y="Ki") -> (x*y=w124:dbl)
        "Ki part" <- w124
        n155 = Bundle "捆绑"("cx"=w53, "cy"=w51) -> (w74:cluster{"cx":ext, "cy":ext})  [unwired: 1 in]
        n156 = Compound Arithmetic op=ADD(w136, w131, w124) -> (w38:ext)
        "u(t)_y" <- w38
        n157 = Compound Arithmetic op=ADD(w150, w145, w138) -> (w39:ext)
        "u(t)_x" <- w39
        n158 = Build Array (concatenate) "创建数组"(w65, w74) -> (w49:cluster{"cx":ext, "cy":ext}[])
        n159 = Multiply(x="K1", y=w38) -> (x*y=w96:ext)
        "delta_dr" <- w96
        n160 = Multiply(x="k2", y=w39) -> (x*y=w95:ext)
        "delta_pr" <- w95
        n161 = call "IMAQ Overlay Multiple Lines 2"("Image"=w62, "Line End Points"=w49, "Drawing Mode (Frame)"=w73, "Color"=u32 3071, "Width"=u32 5) -> ("Image Out"=→"彩色轨迹":T1)  [unwired: 9 in, 1 out]
        n162 = case shown="真" "打开彩色点轨迹" {
          tunnel: [_ w306] -> w48
          tunnel: w49 -> [_ w306]
          frame False {
          }
          frame True {
          }
        }
        n163 = feedback-in #6(w106) -> ()
        n164 = feedback-in #7(w113) -> ()
        n165 = Multiply(x=w106, y=0.6) -> (x*y=w102:dbl)
        n166 = Multiply(x=w113, y=0.6) -> (x*y=w109:dbl)
        n167 = Add(x=w102, y=w101) -> (x+y=w99:dbl)
        "MLP_pr" <- w99
        n168 = Add(x=w95, y=w99) -> (x+y=w97:ext)
        "magnet_input_pr" <- w97
        n169 = Add(x=w109, y=w108) -> (x+y=w100:dbl)
        "MLP_dr" <- w100
        n170 = Add(x=w96, y=w100) -> (x+y=w98:ext)
        "magnet_input_dr" <- w98
        n171 = case shown="\"Rotating Field\", 默认" "Parameter Settings" {
          tunnel: w303 -> [w319 w334 w349 w368 w387 w401 w419 w434]
          tunnel: w302 -> [w316 w333 w348 w367 w385 w400 w417 w433]
          tunnel: [w318 w332 w346 w366 w386 w399 w418 w432] -> w301
          tunnel: [w317 w331 w347 w365 w384 w398 w416 w431] -> w300
          tunnel: [w312 w325 w340 w361 w378 w393 w414 w426] -> w299
          tunnel: "Pause" -> [w310 w323 w338 w360 w377 w392 w409 w424]
          tunnel: [_ _ _ w357 _ _ _ _] -> w235
          tunnel: [_ _ _ w358 _ _ _ _] -> w233
          tunnel: w153 -> [_ _ _ w356 _ _ _ _]
          tunnel: [_ _ _ w355 _ _ _ _] -> w167
          tunnel: w98 -> [_ _ _ w354 _ _ _ _]
          tunnel: w97 -> [_ _ _ w353 _ _ _ _]
          frame "Gradient Field " {
            n172 = case shown="假" w310 {
              tunnel: ["Ag" 0.0] -> w311
              frame False {
              }
              frame True {
              }
            }
            n173 = Build Array(1.0, w311, "pg", "dg", "fg") -> (w312:dbl[])
            n174 = shared-variable-write(w319, w316, w312, 1000 ("timeout ms (-1)")) -> (w318:refnum<k21>, w317:errorcluster)  [unwired: 1 out]
          }
          frame "Oscillating Field" {
            n175 = case shown="假" w323 {
              tunnel: ["AoOF" 0.0] -> w324
              frame False {
              }
              frame True {
              }
            }
            n176 = Build Array(2.0, w324, "oo", "fo", "po", "do") -> (w325:dbl[])
            n177 = shared-variable-write(w334, w333, w325, 1000 ("timeout ms (-1)")) -> (w332:refnum<k21>, w331:errorcluster)  [unwired: 1 out]
          }
          frame "Conical Field" {
            # "FG"
            n178 = case shown="假" w338 {
              tunnel: ["Ac" 0.0] -> w339
              frame False {
              }
              frame True {
              }
            }
            n179 = Build Array(3.0, w339, "wc", "pc", "dc", "cc") -> (w340:dbl[])
            n180 = shared-variable-write(w349, w348, w340, 1000 ("timeout ms (-1)")) -> (w346:refnum<k21>, w347:errorcluster)  [unwired: 1 out]
          }
          frame "Rotating Field", Default {
            n181 = case shown="假" w360 {
              tunnel: ["Ar" 0.0] -> w357
              frame False {
              }
              frame True {
              }
            }
            n182 = case shown="真" "磁场变换" {
              tunnel: [sgl 0.0 ("pr") w372] -> w363
              tunnel: [sgl 0.0 ("dr") w373] -> w358
              tunnel: w356 -> [_ w374]
              tunnel: [_ w372] -> w355
              tunnel: w354 -> [_ w373]
              tunnel: w353 -> [_ w372]
              frame False {
              }
              frame True {
                n183 = formula code="int p;\n    int q;\n    q = t/50 ;  \n    p = q%36; //用来构造循环\n    dr = -180 + (p*10);\n\n    int p2;\n    int q2;\n    q2 = q/(72);\n    p2 = q2%36; //用来构造循环\n    pr =  -40 + p2*10;"("t"=w374) -> ()  [unwired: 2 out]
                "dr" <- w373
                "pr" <- w372
              }
            }
            n184 = Build Array(4.0, w357, "wr", w363, w358) -> (w361:ext[])
            n185 = shared-variable-write "向流中写入单个元素"(w368, w367, w361, 1000 ("timeout ms (-1)")) -> (w366:refnum<k21>, w365:errorcluster)  [unwired: 1 out]
          }
          frame "Disassembly" {
            n186 = case shown="假" w377 {
              tunnel: ["Dis strength(mT)" 0.0] -> w382
              frame False {
              }
              frame True {
              }
            }
            n187 = Build Array(5.0, w382, "Dis tumbling frequency (Hz)", "Dis phase frequency (Hz)", "Dis phase step") -> (w378:dbl[])
            n188 = shared-variable-write(w387, w385, w378, 1000 ("timeout ms (-1)")) -> (w386:refnum<k21>, w384:errorcluster)  [unwired: 1 out]
          }
          frame "Swarm" {
            n189 = case shown="假" w392 {
              tunnel: ["Swa strength (mT)" 0.0] -> w391
              frame False {
              }
              frame True {
              }
            }
            n190 = Build Array(6.0, w391, "Swa frequency (Hz)", "Swa pitch angle (deg)", "Swa direction angle (deg)", "Swa ratio") -> (w393:dbl[])
            n191 = shared-variable-write(w401, w400, w393, 1000 ("timeout ms (-1)")) -> (w399:refnum<k21>, w398:errorcluster)  [unwired: 1 out]
          }
          frame "Ribbon Oscillating Field" {
            n192 = case shown="假" w409 {
              tunnel: ["Strength (mT)" 0.0] -> w408
              frame False {
              }
              frame True {
              }
            }
            n193 = Build Array(7.0, w408, "Frequency (Hz)", "Ratio (A/C)", "Direction Angle (deg)", "Pitch Angle (rotating around Origin, deg)", "Pitch Angle (rotating around Constant, deg)") -> (w414:dbl[])
            n194 = shared-variable-write(w419, w417, w414, 1000 ("timeout ms (-1)")) -> (w418:refnum<k21>, w416:errorcluster)  [unwired: 1 out]
          }
          frame "Elliptical Field" {
            n195 = case shown="假" w424 {
              tunnel: ["Ar 2" 0.0] -> w425
              frame False {
              }
              frame True {
              }
            }
            n196 = Build Array(8.0, w425, "wr  2", "pr  2", "dr  2", "ratio", "p_x") -> (w426:dbl[])
            n197 = shared-variable-write(w434, w433, w426, 1000 ("timeout ms (-1)")) -> (w432:refnum<k21>, w431:errorcluster)  [unwired: 1 out]
          }
        }
        "Array" <- w299
        "场强" <- w235
        "dr" <- w233
        n198 = Build Array (concatenate)(w232, w233) -> (w229:ext[])
        "direction angle" <- w229
        n199 = Build Array (concatenate)(w166, w167) -> (w165:ext[])
        n200 = Build Array (concatenate)(w234, w235) -> (w230:dbl[])
        "strength" <- w230
        n201 = Or(x=w300, y="Stop") -> (x .or. y?=w296:bool)
        n202 = Build Array(w231, w230, w229, w228, w223, w227, w226, w225, w219, w215, w196, w195, w182, w178, w173, w165) -> (→"all parameters":ext[][])
        "Numeric 5" <- w153
        "T" <- w153
        "T" <- w153
        "prev_end_point_x" <- w211
        "prev_end_point_y" <- w207
        "prev time" <- w190
      }
    }
    frame #3 {
      # "4. The error -314220 indicates that the other endpoint has been destroyed. The VI ignores this error."
      # "3. Destroy the stream endpoint when you click Stop or when an error occurs."
      # "Close"
      n203 = Flush Stream(8:w444, 11:w447) -> (0:w445:errorcluster, 3:w446:refnum<k21>)  [unwired: 2 in, 1 out]
      n204 = Destroy Stream Endpoint(8:w445, 11:w446) -> (0:w439:errorcluster)
      n205 = Unbundle By Name(w439) -> ("code"=w443:i32)
      n206 = xnode "Error Ring"() -> ("错误输出"=w440:errorcluster)
      n207 = Not Equal?(x=w443, y=-314220) -> (x != y?=w441:bool)
      n208 = Select(t=w439, s=w441, f=w440) -> (s? t:f=→"error out":errorcluster)
    }
  }
